vi "Raise.vi"(5 "Message":string, 7 "Code":i32, 8 "error in (no error)":errorcluster, 11 "Error in":refnum<class "Error.lvclass">) -> (0 "error out":errorcluster, 3 "Error out":refnum<class "Error.lvclass">)   [LabVIEW 2022 SP3, in "Error.lvlib" / "Error.lvclass"]
uses:
  Error.lvclass
  Error.lvclass/Error.ctl
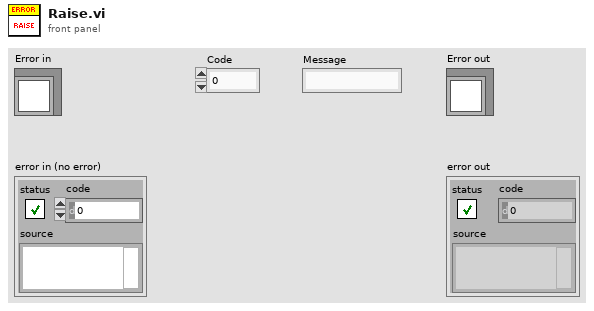
[diagram p1: front panel]
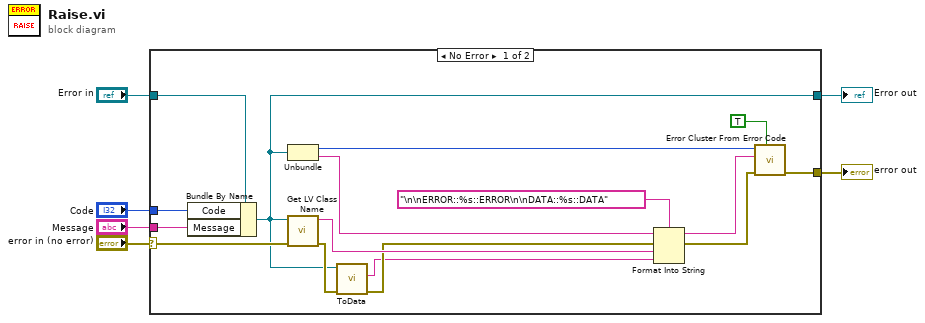
[diagram p0: block diagram]
diagram:
  n1 = case shown="No Error" "error in (no error)" {
    selector: "error in (no error)" -> [w22 w24]
    tunnel: [w20 w24] -> w5
    tunnel: [w11 w23] -> w3
    tunnel: "Error in" -> [w7 w23]
    tunnel: "Code" -> [w9 _]
    tunnel: "Message" -> [w8 _]
    frame No Error {
      n2 = Bundle By Name(cluster=w7, "Code"=w9, "Message"=w8) -> (w11:refnum<class "Error.lvclass">)
      n3 = Unbundle(w11) -> (w21:i32, w15:string)
      n4 = call <vilib>:"Get LV Class Name.vi"("error in (no error)"=w22, "object"=w11) -> ("error out"=w13:errorcluster, "class name"=w16:string)  [unwired: 8 in]
      n5 = call-dynamic "ToData.vi"("error in (no error)"=w13, "Error in"=w11) -> ("error out"=w12:errorcluster, "Data"=w10:string)  [unwired: 7 in, 1 out]
      n6 = Format Into String(format string="\n\nERROR::%s::ERROR\n\nDATA::%s::DATA", initial string=w15, error in=w12, w16, w10) -> (resulting string=w14:string, error out=w18:errorcluster)
      n7 = call <vilib>:"Error Cluster From Error Code.vi"("show call chain? (False)"=TRUE, "error in (no error)"=w18, "error message (\"\")"=w14, "error code (0)"=w21) -> ("error out"=w20:errorcluster)  [unwired: 5 in]
    }
    frame Error {
    }
  }
  "error out" <- w5
  "Error out" <- w3
